vi "UpdateBaseActor.vi"(10 "VIRef":refnum<vi>, 11 "Actor":refnum<class "Actor.lvclass">) -> (3 "Actor":refnum<class "Actor.lvclass">)   [LabVIEW 2025]
uses:
  Actor/Actor.lvclass
  Message.ctl
  Message/Message.lvclass
  jettl.lvlib
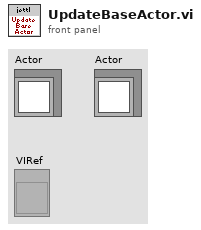
[diagram p1: front panel]
types:
  T1 = typedef "jettl.lvlib/BaseActor.ctl" = cluster{"Lifetime":T2, "SelfActor":T3, "MediatorActor":T3, "ComponentActorMap":T8}
  T2 = typedef "jettl.lvlib/Lifetime.ctl" = enum16{"Init", "Spawn", "Setup", "TeardownBeforeRunning", "Running", "StopCalled", "StoppingWithComponents", "StoppingNoComponents", "TeardownAfterRunning", "Stopped"}
  T3 = typedef "jettl.lvlib/Actor.ctl" = cluster{"Messages":T4, "ActorAlias":string, "ActorType":T7, "Transport":refnum<user-event>, "VIRef":refnum<vi>}
  T4 = typedef "jettl.lvlib/Messages.ctl" = cluster{"Listen":T5, "TellSelf":T5, "TellMediator":T5, "TellComponentMap":T6}
  T5 = typedef "jettl.lvlib/MessageSet.ctl" = set{refnum<class "Message.lvclass">}
  T6 = typedef "jettl.lvlib/TellComponentMap.ctl" = map{string, T5}
  T7 = typedef "jettl.lvlib/ActorType.ctl" = enum16{"Mediator", "Component"}
  T8 = typedef "jettl.lvlib/ComponentActorMap.ctl" = map{string, T3}
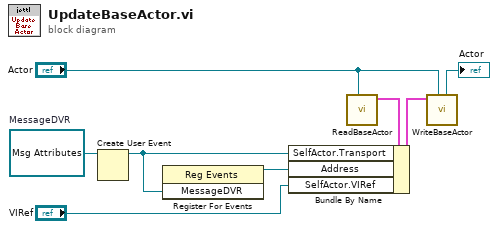
[diagram p0: block diagram]
diagram:
  w7 = refnum<data-value> refnum  # MessageDVR
  n1 = Create User Event(user event datatype=w7) -> (user event=w6:refnum<user-event>)  [unwired: 1 in, 1 out]
  n2 = register-events(w6) -> (reference out=w5:refnum<event-registration>)  [unwired: 2 in, 1 out]
  n3 = call-dynamic "ReadBaseActor.vi"("Actor"="Actor") -> ("BaseActor"=w2:T1)  [unwired: 10 in]
  n4 = Bundle By Name(cluster=w2, "SelfActor.Transport"=w6, "Address"=w5, "SelfActor.VIRef"="VIRef") -> (w1:T1)
  n5 = call-dynamic "WriteBaseActor.vi"("Actor"="Actor", "BaseActor"=w1) -> ("Actor"=→"Actor":refnum<class "Actor.lvclass">)  [unwired: 9 in]
